vi "Host - Get Third Party ECAT IOVs.vi"(0 "ECAT Slave in":refnum<k21>="ni.var.io:/", 11 "error in (no error)":errorcluster) -> (4 "ECAT Slave out":refnum<k21>="ni.var.io:/", 6 "ECAT Modules":refnum<k21>[](array[refnum]), 8 "ECAT Variablenobjekt":refnum<k21>[](array[refnum]), 15 "error IO":errorcluster)   [LabVIEW 2020, in "SEECD System Explorer.lvlib"]
uses:
  SEECD System Explorer.lvlib
  <resource>/objmgr/IndComECAT.rc
  <vilib>/regexp/Match Regular Expression.xnode
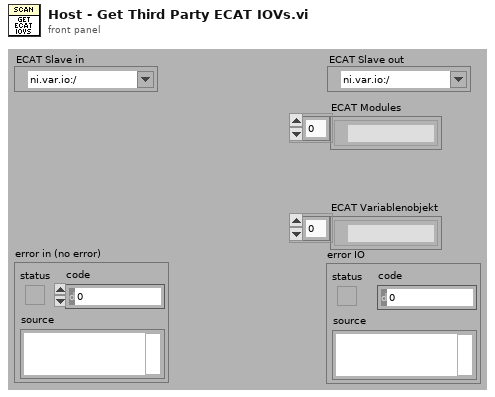
[diagram p1: front panel]
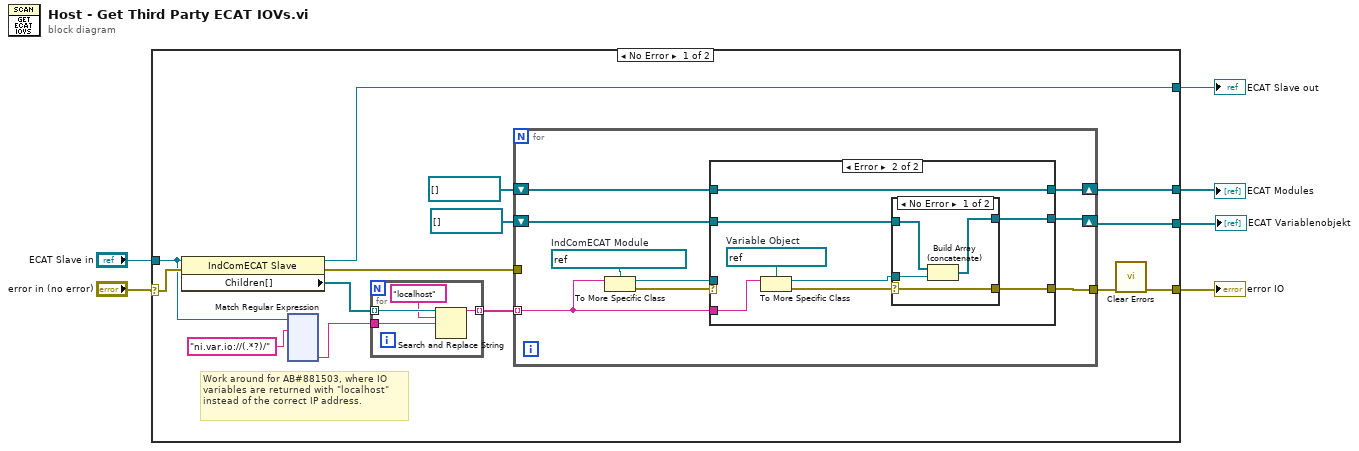
[diagram p0: block diagram]
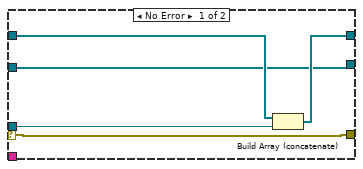
[diagram p2: hidden frame]
diagram:
  n1 = case shown="No Error" "error in (no error)" {
    selector: "error in (no error)" -> [w18 w170]
    tunnel: [w20 w170] -> w6
    tunnel: "ECAT Slave in" -> [w8 w169]
    tunnel: [w19 w169] -> w4
    tunnel: [w14 _] -> w2
    tunnel: [w12 _] -> w1
    frame No Error {
      # "Work around for AB#881503, where IO variables are returned with \"localhost\" instead of the correct IP address."
      n2 = property class="IndComECAT Slave"(reference=w8, error in=w18) -> (reference out=w19:refnum<k21>, error out=w17:errorcluster, "Children[]"=w11:refnum<k21>[])
      n3 = xnode "Match Regular Expression"("input string"=w8, "regular expression"="ni.var.io://(.*?)/" ("format string")) -> ("submatch 1"=w7:string)  [unwired: 4 in, 5 out]
      n4 = for {
        tunnel: w11 -> [w52] mode=indexing
        tunnel: [w51] -> w10 mode=indexing
        tunnel: w7 -> [w50]
        n5 = Search and Replace String(input string=w52, search string="localhost", replace string=w50) -> (result string=w51:string)  [unwired: 5 in, 3 out]
      }
      n6 = for {
        tunnel: w10 -> [w26] mode=indexing
        tunnel: w17 -> [_]
        tunnel: [w29] -> w16
        shift-right: [w27] -> w14
        shift-left: refnum<k21>[] [] -> [w28]
        shift-right: [w24] -> w12
        shift-left: refnum<k21>[] [] -> [w25]
        w23 = refnum<k21> refnum  # IndComECAT Module
        n7 = To More Specific Class(target class=w23, reference=w26) -> (specific class reference=w21:refnum<k21>, error out=w22:errorcluster)  [unwired: 1 in]
        n8 = case shown="Error" w22 {
          selector: w22 -> [w32 _]
          tunnel: [w33 w36] -> w27
          tunnel: w21 -> [w34 _]
          tunnel: [w32 w35] -> w29
          tunnel: w28 -> [w31 w36]
          tunnel: w26 -> [_ w41]
          tunnel: w25 -> [w30 w38]
          tunnel: [w30 w37] -> w24
          frame No Error {
            n9 = Build Array (concatenate)(w31, w34) -> (w33:refnum<k21>[])
          }
          frame Error {
            w42 = refnum<k21> refnum  # Variable Object
            n10 = To More Specific Class(target class=w42, reference=w41) -> (specific class reference=w39:refnum<k21>, error out=w40:errorcluster)  [unwired: 1 in]
            n11 = case shown="No Error" w40 {
              selector: w40 -> [w43 w48]
              tunnel: [w46 w47] -> w37
              tunnel: w39 -> [w45 _]
              tunnel: w38 -> [w44 w47]
              tunnel: [w43 w48] -> w35
              frame No Error {
                n12 = Build Array (concatenate)(w44, w45) -> (w46:refnum<k21>[])
              }
              frame Error {
              }
            }
          }
        }
      }
      n13 = call <vilib>:"Clear Errors.vi"("error in (no error)"=w16) -> ("error out"=w20:errorcluster)  [unwired: 5 in, 1 out]
    }
    frame Error {
    }
  }
  "error IO" <- w6
  "ECAT Slave out" <- w4
  "ECAT Modules" <- w2
  "ECAT Variablenobjekt" <- w1
